vi "PIDController_Pack_AdvTuning.vi"(0 "Filter Derivative":bool, 4 "MinimumIntegral":dbl=-9.9e+30, 5 "Kn":dbl=1.0, 6 "MaximumIntegral":dbl=9.9e+30, 7 "Kf":dbl, 9 "Kd":dbl, 10 "Ki":dbl, 11 "Kp":dbl) -> (3 "Adv PID Tuning":T1={"Kf"=0.0, "Kp"=0.0, "Ki"=0.0, "Kd"=0.0, "MaximumIntegral"=9.9e+30, "MinimumIntegral"=-9.9e+30, "Filter Derivative"=FALSE})   [LabVIEW 2019, in "Trajectory_Library.lvlib"]
doc: "Convience function to pack individual tuning parameter values into a cluster to pass to the Advanced PID controller\n\nInputs:\n - Kn -- Optional normalizing constants. When present, the other constants are multiplied by this constant. Set this equal to the maximum controller output divided by the corresponding maximum process value that corresponds to the maximum controller output. Using this can help simlify tuning.\n - Kf -- Feedforward gain constant. The feedforward value is multiplied by this value. Generally this translates the units of the input to the units of the output. (For example if a drive maximum speed is 10 FT/SEC, when the motor output is 1.0, this gain can be set to 0.1.)\n - Kp -- Proportional gain constant. The error is multiplied by this value. (Default = 0.0)\n - Ki -- Integral gain constant. The integral of the error is multiplied by this value. (Default = 0.0)\n - Kd -- Derivative gain constant The derivative of the error is multipled by this value. (Default = 0.0)\n - Maximum Integral -- The integral component of the output is not allowed to exceed this value This limits the travel of the integral This is in units of the output value. ( Default = 9.9E+30 )\n - Minimal Integral -- The integral component of the output is not allowed to be less than this value. This limits the travel of the integral. This is in units of the output value. ( Default = -9.9E+30 )\n - Filter Derivative -- Taking a derivative of the error amplifies the noise in this signal When this boolean is TRUE, the error value used to calculate the derivative portion of the output is passed through a 3 sample average filter.\n\nOutput:\n - Adv PID Tuning -- Cluster containing the tuning values."
uses:
  Trajectory_Library.lvlib
  TypeDef/PID_ADV_TUNING.ctl
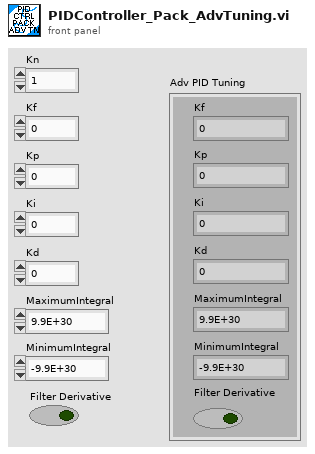
[diagram p1: front panel]
types:
  T1 = typedef "Trajectory_Library.lvlib/PID_ADV_TUNING.ctl" = cluster{"Kf":dbl, "Kp":dbl, "Ki":dbl, "Kd":dbl, "MaximumIntegral":dbl, "MinimumIntegral":dbl, "Filter Derivative":bool}
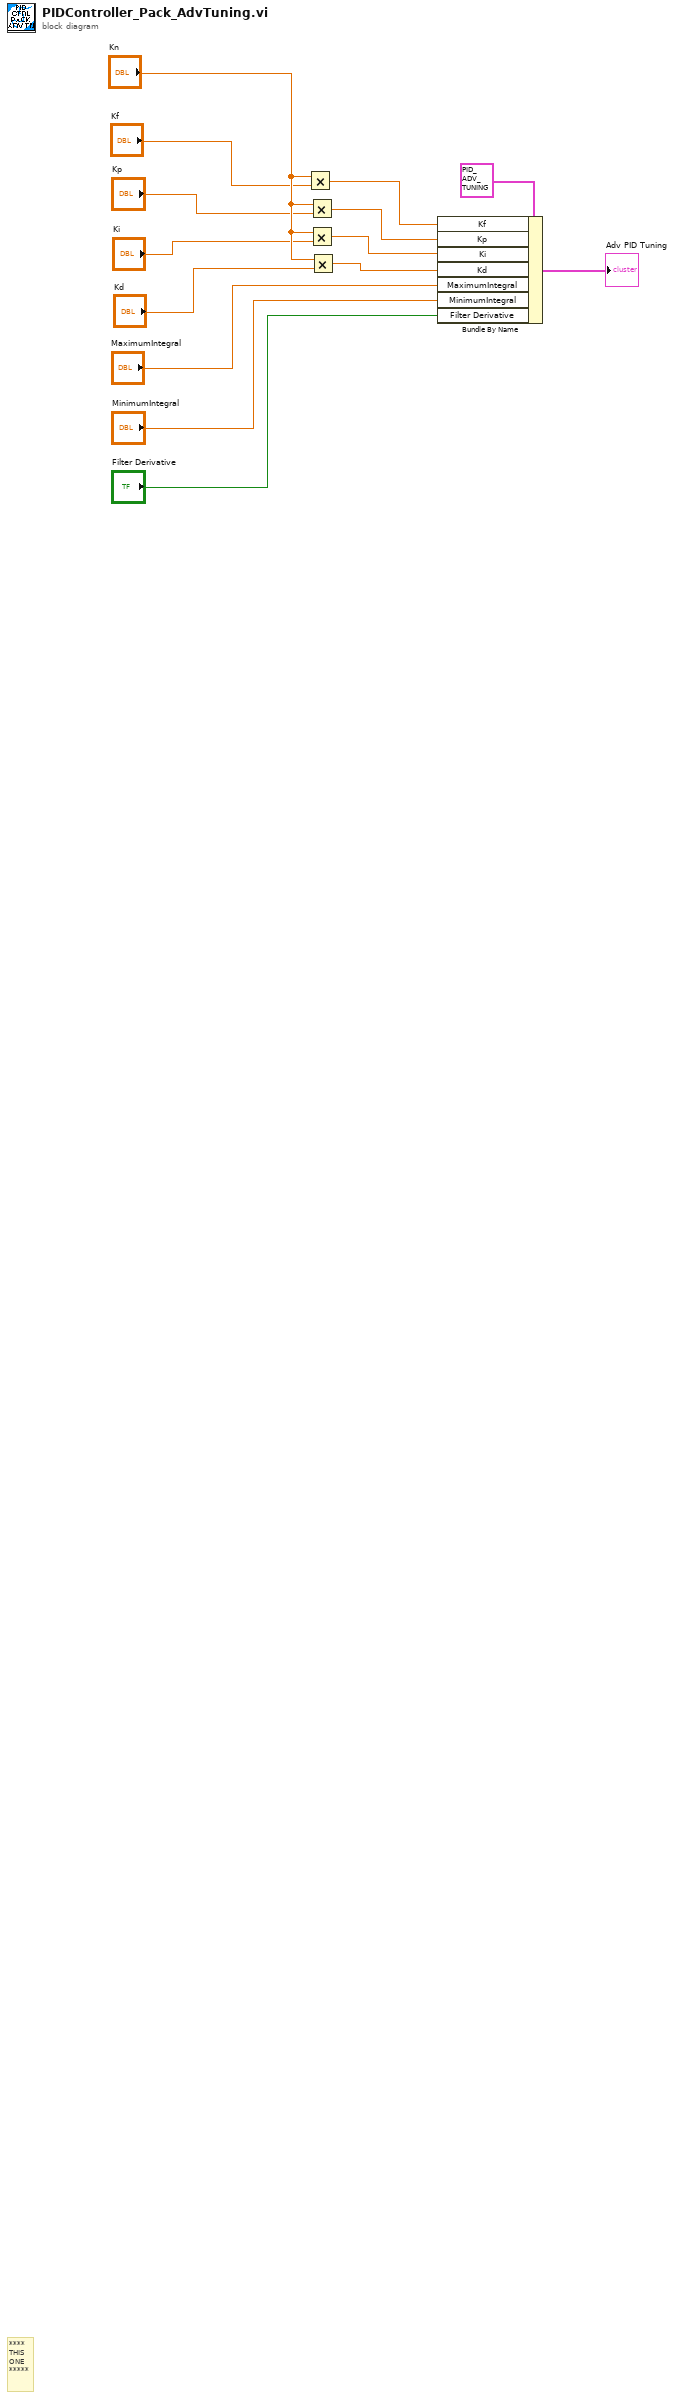
[diagram p0: block diagram]
diagram:
  # "****\nTHIS\nONE\n*****"
  n1 = Multiply(x="Kn", y="Kf") -> (x*y=w6:dbl)
  n2 = Multiply(x="Kn", y="Kp") -> (x*y=w7:dbl)
  n3 = Multiply(x="Kn", y="Ki") -> (x*y=w8:dbl)
  n4 = Multiply(x="Kn", y="Kd") -> (x*y=w9:dbl)
  n5 = Bundle By Name(cluster=T1 {"Kf"=0.0, "Kp"=0.0, "Ki"=0.0, "Kd"=0.0, "MaximumIntegral"=9.9e+30, "MinimumIntegral"=-9.9e+30, "Filter Derivative"=FALSE} ("Adv PID Tuning"), "Kf"=w6, "Kp"=w7, "Ki"=w8, "Kd"=w9, "MaximumIntegral"="MaximumIntegral", "MinimumIntegral"="MinimumIntegral", "Filter Derivative"="Filter Derivative") -> (→"Adv PID Tuning":T1)
